vi "SSC Digital Filter Sites.vi"(0 "Digital SSC In":T1[](array[typedef]), 5 "Desired Sites":i32[](array[numeric])) -> (4 "Digital SSC Out with requested sites":T1[](array[typedef]))   [LabVIEW 2020]
doc: "Filters Digital SSC sessions based on the specified list of desired sites. \n\nNOTE: Once sessions have been filtered, they become separated from their original TSM context and cannot be properly published using pin query context."
uses:
  SSC Digital.ctl
  Shared SubVIs/Site List to Site Numbers.vi
  Shared SubVIs/Channel List to Pins.vi
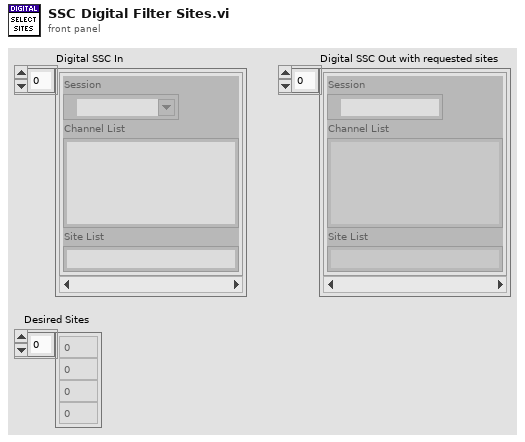
[diagram p1: front panel]
types:
  T1 = typedef "SSC Digital.ctl" = cluster{"Session":refnum<k15>, "Channel List":string, "Site List":string}
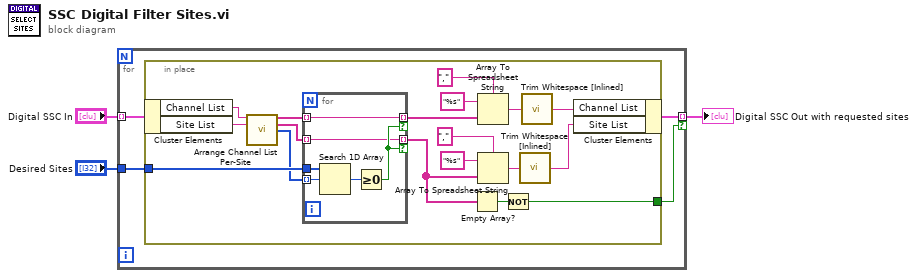
[diagram p0: block diagram]
diagram:
  n1 = for {
    tunnel: "Digital SSC In" -> [w7] mode=indexing
    tunnel: "Desired Sites" -> [w4]
    tunnel: [w6] -> w1 mode=indexing if=w5
    n2 = in-place {
      in-place-border: w4 -> [w23]
      in-place-border: [w9] -> w5
      n3 = in-place-cluster #1(w7) -> ("Channel List"=w25:string, "Site List"=w24:string)
      n4 = call "Arrange Channel List Per-Site.vi"("Channel List String"=w25, "Site List String"=w24) -> ("Channel List Array"=w21:string[], "Site List Array"=w20:string[], "Site Numbers"=w22:i32[])  [unwired: 11 in]
      n5 = for {
        tunnel: w21 -> [w29] mode=indexing
        tunnel: w22 -> [w28] mode=indexing
        tunnel: w23 -> [w31]
        tunnel: [w29] -> w11 mode=indexing if=w27
        tunnel: [w26] -> w8 mode=indexing if=w27
        tunnel: w20 -> [w26] mode=indexing
        n6 = Search 1D Array(1D array=w31, element=w28) -> (index of element=w30:i32)  [unwired: 1 in]
        n7 = Greater Or Equal To 0?(x=w30) -> (x >= 0?=w27:bool)
      }
      n8 = Empty Array?(array=w8) -> (empty?=w10:bool)
      n9 = Array To Spreadsheet String(delimiter (Tab)=",", array=w11, 3:"%s" ("format string")) -> (spreadsheet string=w15:string)
      n10 = Array To Spreadsheet String(delimiter (Tab)=",", array=w8, 3:"%s" ("format string")) -> (spreadsheet string=w13:string)
      n11 = Not(x=w10) -> (.not. x?=w9:bool)
      n12 = call "Trim Whitespace [Inlined].vi"("string"=w13) -> ("trimmed string"=w12:string)  [unwired: 1 in]
      n13 = call "Trim Whitespace [Inlined].vi"("string"=w15) -> ("trimmed string"=w14:string)  [unwired: 1 in]
      n14 = in-place-cluster #1("Channel List"=w14, "Site List"=w12) -> (w6:T1)
    }
  }
  "Digital SSC Out with requested sites" <- w1
